vi "GetDeterministicGuid.vi"(8 "error in":errorcluster, 11 "FilePath":path) -> (0 "error out":errorcluster, 3 "GUID":string)   [LabVIEW 2021, in "ProligentXMLGenerator.lvlib" / "Document.lvclass"]
uses:
  Document.lvclass
  <vilib>/security/Message Digest/API/Instances/File/SHA-256 File Checksum.vi
  Document.lvclass/Document.ctl
  <vilib>/security/Message Digest/API/NI_Message Digest API.lvlib
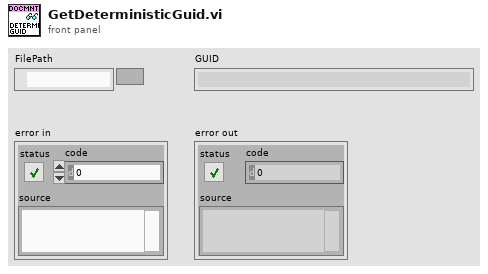
[diagram p1: front panel]
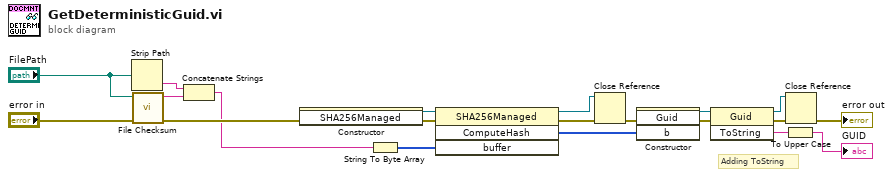
[diagram p0: block diagram]
diagram:
  # "Adding ToString"
  n1 = Strip Path(path="FilePath") -> (name=w5:string)  [unwired: 1 out]
  n2 = call-poly <vilib>:"File Checksum.vi"("error in"="error in", "path"="FilePath") -> ("error out"=w7:errorcluster, "digest"=w6:string)  [unwired: 8 in]
  n3 = Concatenate Strings(w5, w6) -> (w4:string)
  n4 = constructor class="SHA256Managed"(error in=w7) -> (reference out=w20:refnum<k24>, error out=w18:errorcluster)  [unwired: 2 in, 1 out]
  n5 = String To Byte Array(string=w4) -> (unsigned byte array=w19:u8[])
  n6 = invoke class="SHA256Managed" method="ComputeHash"(reference=w20, error in=w18, "buffer"=w19) -> (reference out=w1:refnum<k24>, error out=w17:errorcluster, "ComputeHash"=w14:u8[])  [unwired: 1 in, 1 out]
  n7 = Close Reference(reference=w1, error in (no error)=w17) -> (error out=w9:errorcluster)
  n8 = constructor class="Guid"(error in=w9, "b"=w14) -> (reference out=w15:refnum<k24>, error out=w16:errorcluster)  [unwired: 2 in, 2 out]
  n9 = invoke class="Guid" method="ToString"(reference=w15, error in=w16) -> (reference out=w10:refnum<k24>, error out=w11:errorcluster, "ToString"=w13:string)  [unwired: 1 in]
  n10 = To Upper Case(1:w13) -> (0:→"GUID":string)
  n11 = Close Reference(reference=w10, error in (no error)=w11) -> (error out=→"error out":errorcluster)
